vi "Do.vi"(8 "error in (no error)":errorcluster, 10 "Actor in":refnum<class "Actor.lvclass">, 11 "Load App Msg in":refnum<class "Load App Msg.lvclass">) -> (0 "error out":errorcluster, 2 "Actor out":refnum<class "Actor.lvclass">)   [LabVIEW 2018, in "MWWL Verification.lvlib" / "Load App Msg.lvclass"]
doc: "(<B>Filename</B>: Actor Framework.lvlib:Message.lvclass:Do.vi)\n\nDefines what a message does when it is received by an actor. Generally, a message instructs an actor to invoke one of its methods. By default, this method does nothing. A child class must override it to define behavior. Create a child class by using the Actor Framework Message Maker dialog box."
uses:
  Load App Msg.lvclass
  <vilib>/ActorFramework/Actor/Actor.lvclass
  MWWL Verification/MWWL Verification.lvclass
  C:/Program Files (x86)/National Instruments/LabVIEW 2018/vi.lib/ActorFramework/Actor/Actor.lvclass
  Load App Msg.lvclass/Load App Msg.ctl
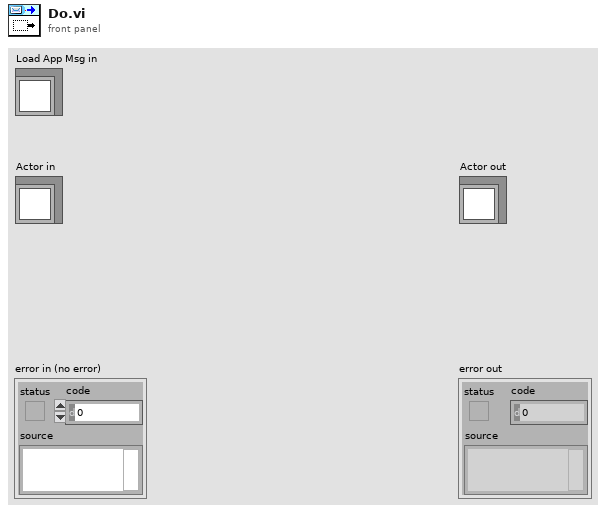
[diagram p1: front panel]
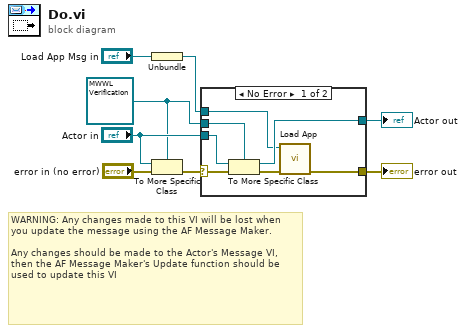
[diagram p0: block diagram]
diagram:
  w3 = refnum<class "MWWL Verification.lvclass"> refnum ("Actor Type")
  # "WARNING: Any changes made to this VI will be lost when you update the message using the AF Message Maker.\n\nAny changes should be made to the Actor's Message VI, then the AF Message Maker's Update function should be used to update this VI"
  n1 = Unbundle("Load App Msg in") -> (w2:refnum<notifier>)
  n2 = To More Specific Class(target class=w3, reference="Actor in", error in="error in (no error)") -> (error out=w7:errorcluster)  [unwired: 1 out]
  n3 = case shown="No Error" w7 {
    selector: w7 -> [w15 w17]
    tunnel: [w11 w17] -> w6
    tunnel: [w10 w16] -> w5
    tunnel: "Actor in" -> [w14 w16]
    tunnel: w3 -> [w13 _]
    tunnel: w2 -> [w9 _]
    frame No Error {
      n4 = To More Specific Class ("Actor Cast")(target class=w13, reference=w14, error in=w15) -> (specific class reference=w10:refnum<class "MWWL Verification.lvclass">, error out=w12:errorcluster)
      n5 = call "Load App.vi"("error in (no error)"=w12, "Status Notifier"=w9) -> ("error out"=w11:errorcluster)  [unwired: 9 in]
    }
    frame Error {
    }
  }
  "error out" <- w6
  "Actor out" <- w5
